vi "Builder.Run.vi"(8 "error in (no error)":errorcluster, 10 "Thread Parameters":refnum<class "Thread Parameters.lvclass">, 11 "Builder in":refnum<class "Builder.lvclass">) -> (0 "error out":errorcluster, 3 "Builder out":refnum<class "Builder.lvclass">)   [LabVIEW 2016, in "DSF.Engine.lvlib" / "Builder.lvclass"]
uses:
  Builder.lvclass
  Thread Parameters/Thread Parameters.lvclass
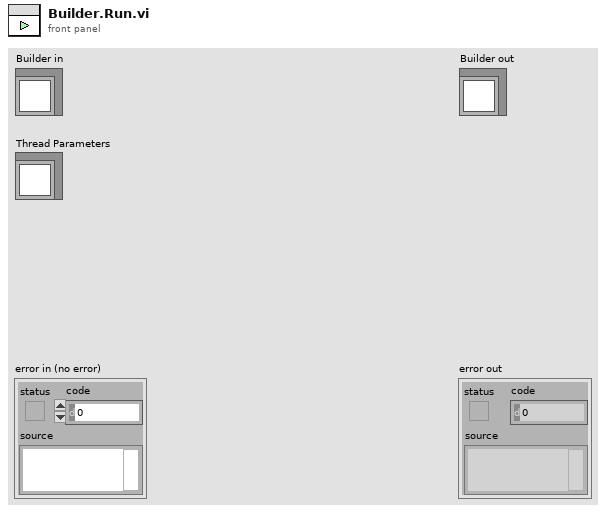
[diagram p1: front panel]
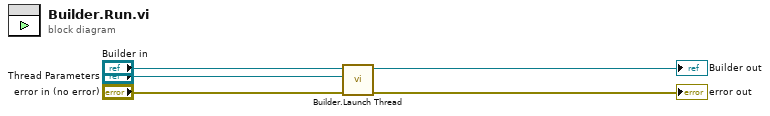
[diagram p0: block diagram]
diagram:
  n1 = call "Builder.Launch Thread.vi"("error in (no error)"="error in (no error)", "Thread Parameters"="Thread Parameters", "Builder in"="Builder in") -> ("error out"=→"error out":errorcluster, "Builder out"=→"Builder out":refnum<class "Builder.lvclass">)  [unwired: 7 in]
